vi "Tacking Helper - Final (First) Tack Point.vi"(6 "Intermediate\nWaypoints In":T2[](array[typedef]), 9 "Angle from boat to waypoint":dbl, 10 "End of Array":i32, 11 "Distance to boat":dbl) -> (3 "Intermediate\nWaypoints Out":T2[](array[typedef]))   [LabVIEW 2011]
doc: "This vi takes a tack pattern along with the leftover distance to the boat, and extrapolates the angle last used to get the last intermediate waypoint. If done as originally intended, this occurs after all of the jumps, is the only point that doesn't contact the bounding box, and is the closest waypoint to the boat.\n\nTO DO: This vi needs to have at least one jump already completed before it will work - it needs to have a prior angle to go off of."
uses:
  <vilib>/Analysis/NI_AAL_Angle.lvlib
  <vilib>/Analysis/coordinate.llb/Absolute Angle Difference (scalar).vi
  0x2-OCU-Think Comm/0x2 Typedefs/waypointTypes.ctl
  2 Typedefs/UTM Location.ctl
  0x2-OCU-Think Comm/0x2 Typedefs/ocuWaypoint.ctl
panel:
  in  "Boat Position 2":T1
  in  "Boat Position":T1
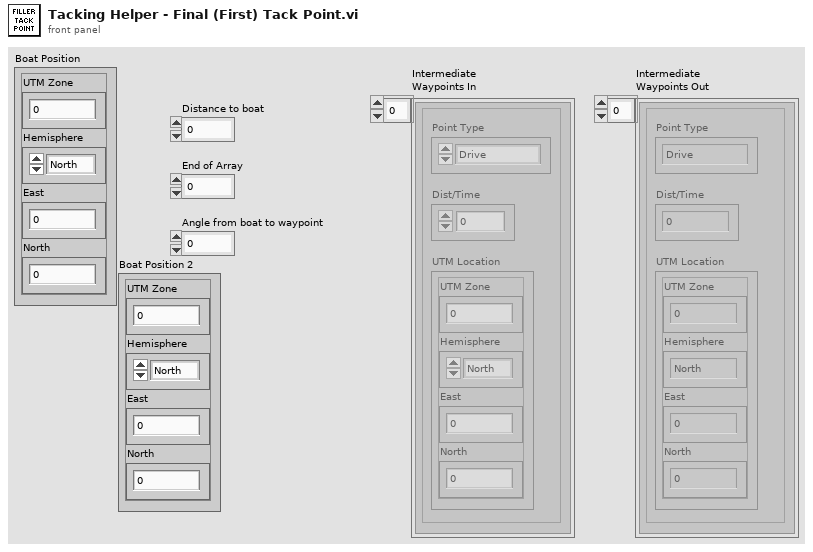
[diagram p1: front panel]
types:
  T1 = typedef "UTM Location.ctl" = cluster{"UTM Zone":dbl, "Hemisphere":enum16{"North", "South"}, "East":dbl, "North":dbl}
  T2 = typedef "ocuWaypoint.ctl" = cluster{"Point Type":T3, "Dist/Time":dbl, "UTM Location":T1}
  T3 = typedef "waypointTypes.ctl" = enum16{"Drive", "Round Port", "Round Starboard", "Stay"}
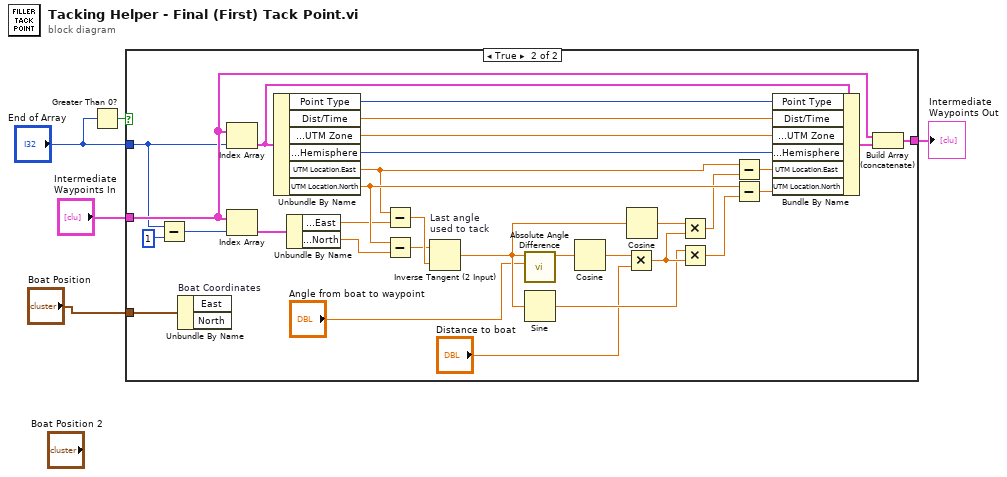
[diagram p0: block diagram]
diagram:
  n1 = Greater Than 0?(x="End of Array") -> (x > 0?=w3:bool)
  n2 = case shown="True" w3 {
    tunnel: [_ w22] -> w5
    tunnel: "Intermediate\nWaypoints In" -> [_ w9]
    tunnel: "End of Array" -> [_ w8]
    tunnel: "Boat Position" -> [_ w6]
    frame False {
    }
    frame True {
      n3 = Subtract(x=w8, y=1) -> (x-y=w17:i32)
      n4 = Unbundle By Name "Boat Coordinates"(w6) -> ()  [unwired: 2 out]
      n5 = Index Array(array=w9, index=w8) -> (element=w10:T2)
      n6 = Index Array(array=w9, index=w17) -> (element=w18:T2)
      n7 = Unbundle By Name(w10) -> ("Point Type"=w12:T3, "Dist/Time"=w13:dbl, "UTM Location.UTM Zone"=w14:dbl, "UTM Location.Hemisphere"=w15:enum16{"North", "South"}, "UTM Location.East"=w35:dbl, "UTM Location.North"=w36:dbl)
      n8 = Unbundle By Name(w18) -> ("UTM Location.East"=w34:dbl, "UTM Location.North"=w7:dbl)
      n9 = Subtract(x=w35, y=w34) -> (x-y=w20:dbl)
      n10 = Subtract(x=w36, y=w7) -> (x-y=w19:dbl)
      n11 = Inverse Tangent (2 Input) "Last angle\nused to tack"(1:w20, 2:w19) -> (0:w26:dbl)
      n12 = call-poly <vilib>:"Absolute Angle Difference.vi"("angle 2"="Angle from boat to waypoint", "angle 1"=w26) -> ("absolute angle difference"=w23:dbl)  [unwired: 8 in, 1 out]
      n13 = Sine(x=w26) -> (sin(x)=w28:dbl)
      n14 = Cosine(x=w23) -> (cos(x)=w24:dbl)
      n15 = Multiply(x=w24, y="Distance to boat") -> (x*y=w29:dbl)
      n16 = Cosine(x=w26) -> (cos(x)=w27:dbl)
      n17 = Multiply(x=w27, y=w29) -> (x*y=w30:dbl)
      n18 = Multiply(x=w28, y=w29) -> (x*y=w31:dbl)
      n19 = Subtract(x=w35, y=w30) -> (x-y=w32:dbl)
      n20 = Subtract(x=w36, y=w31) -> (x-y=w33:dbl)
      n21 = Bundle By Name(cluster=w10, "Point Type"=w12, "Dist/Time"=w13, "UTM Location.UTM Zone"=w14, "UTM Location.Hemisphere"=w15, "UTM Location.East"=w32, "UTM Location.North"=w33) -> (w11:T2)
      n22 = Build Array (concatenate)(w9, w11) -> (w22:T2[])
    }
  }
  "Intermediate\nWaypoints Out" <- w5
